vi "Fit N Gaussians.vi"(10 "Initial Parameters":T1(array[cluster]), 11 "Image In":T2) -> (0 "number of function calls":i32, 1 "Best-Fit Parameters":T1(array[cluster]), 2 "Best-Fit Image":T2, 3 "Image Src (Original)":T2)   [LabVIEW 2011]
uses:
  <vilib>/vision/Image Controls.llb/IMAQ Image.ctl
  <vilib>/gmath/NumericalOptimization/Nonlinear Curve Fit LM bound.vi
  <vilib>/gmath/NI_Gmath.lvlib
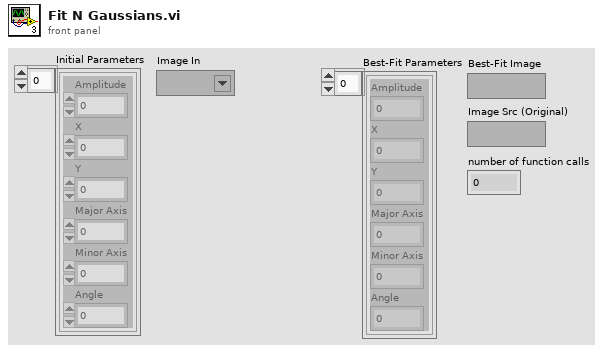
[diagram p1: front panel]
types:
  T1 = cluster{"Amplitude":dbl, "X":dbl, "Y":dbl, "Major Axis":dbl, "Minor Axis":dbl, "Angle":dbl}[]
  T2 = typedef "IMAQ Image.ctl" = refnum<image>
  T3 = typedef "Image Type" = u32
  T4 = cluster{"Width":i32, "Height":i32, "N Gaussians":i32}
  T5 = cluster{"Amplitude":dbl, "X":dbl, "Y":dbl, "Major Axis":dbl, "Minor Axis":dbl, "Angle":dbl}
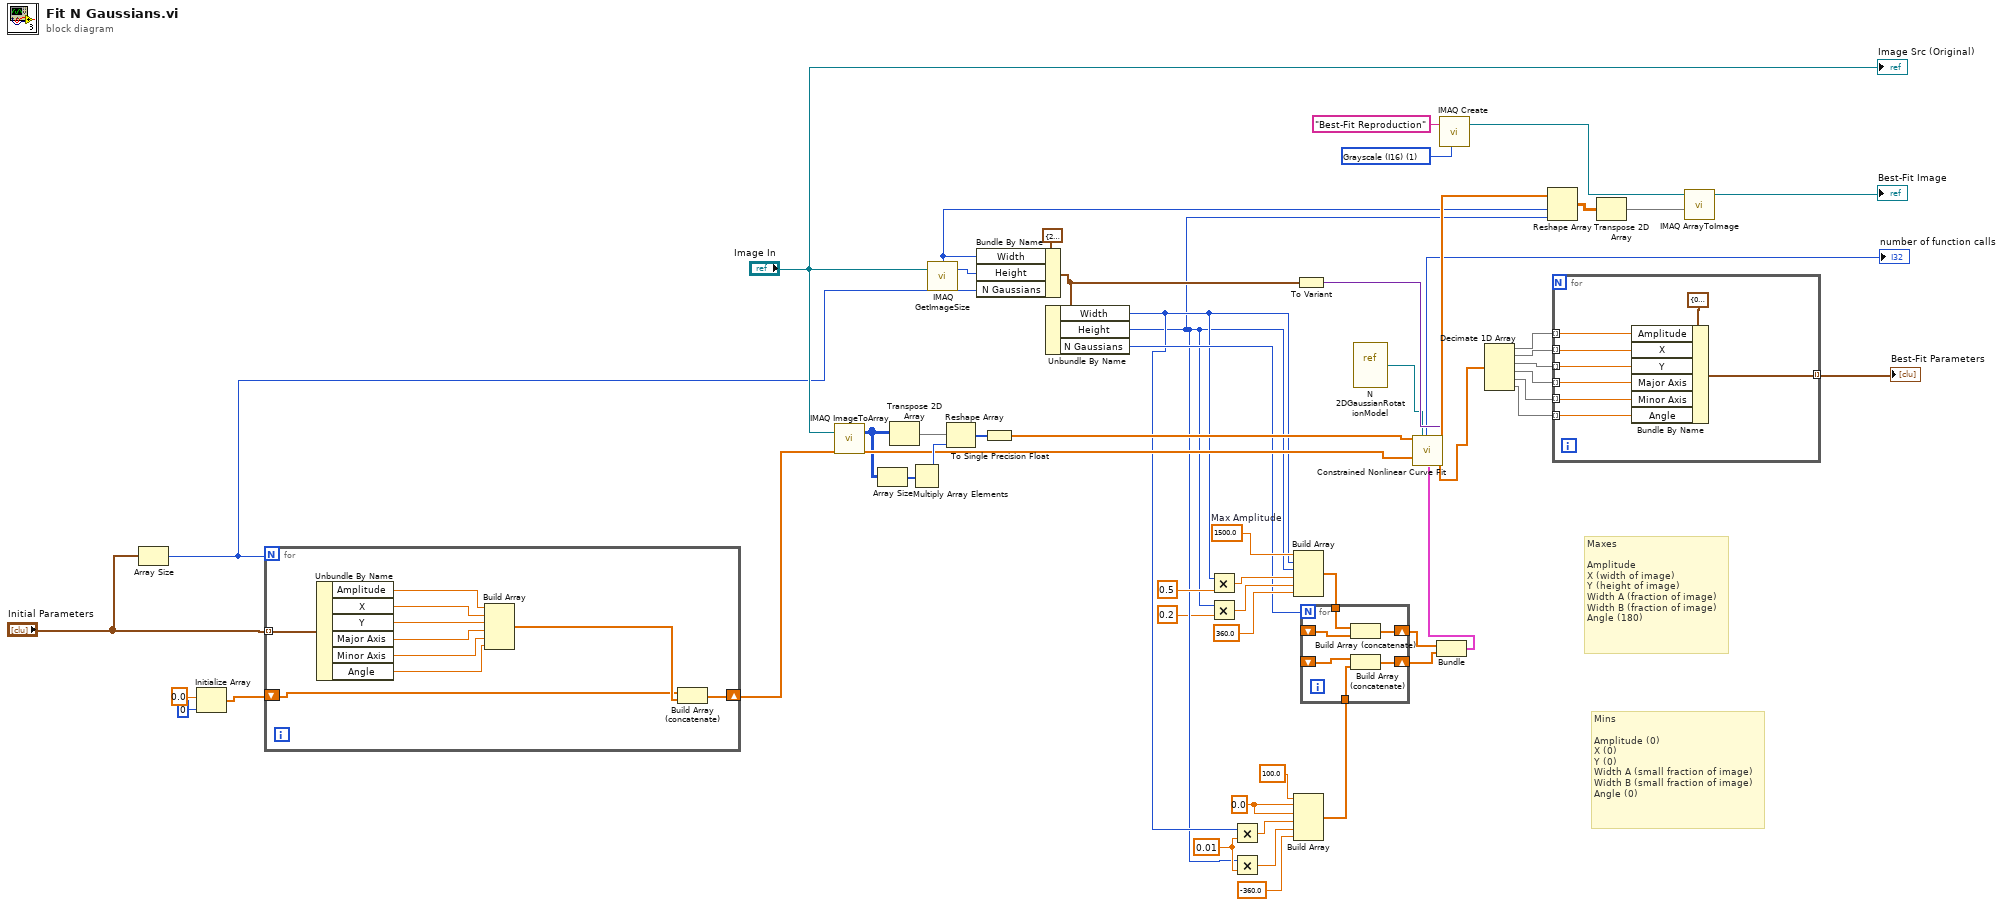
[diagram p0: block diagram]
diagram:
  w25 = 0.01
  w26 = 0.0 ("element")
  w32 = 1500.0  # Max Amplitude
  w43 = T3 1 items=["Grayscale (U8)", "Grayscale (I16)", "Grayscale (SGL)", "Complex (CSG)", "RGB (U32)", "HSL (U32)", "RGB (U64)", "Grayscale (U16)"] ("Image Type")
  # "Mins\n\nAmplitude (0)\nX (0)\nY (0)\nWidth A (small fraction of image)\nWidth B (small fraction of image)\nAngle (0)"
  # "Maxes\n\nAmplitude\nX (width of image)\nY (height of image)\nWidth A (fraction of image)\nWidth B (fraction of image)\nAngle (180)"
  n1 = Array Size(array="Initial Parameters") -> (size(s)=w15:i32)
  n2 = Initialize Array(0.0 ("element"), 0 ("dimension size")) -> (w4:dbl[])
  n3 = for {
    N: w15 -> [_]
    shift-right: [w64] -> w38
    shift-left: w4 -> [w63]
    tunnel: "Initial Parameters" -> [w62] mode=indexing
    n4 = Unbundle By Name(w62) -> ("Amplitude"=w61:dbl, "X"=w60:dbl, "Y"=w59:dbl, "Major Axis"=w58:dbl, "Minor Axis"=w57:dbl, "Angle"=w56:dbl)
    n5 = Build Array(w61, w60, w59, w58, w57, w56) -> (w65:dbl[])
    n6 = Build Array (concatenate)(w63, w65) -> (w64:dbl[])
  }
  n7 = call "IMAQ ImageToArray"("Image"="Image In") -> ("Image Pixels (I16)"=w9:i16[][])  [unwired: 3 in, 4 out]
  n8 = Array Size(array=w9) -> (size(s)=w53:i32[])
  n9 = Transpose 2D Array(2D array=w9) -> (transposed array=w8:i16[][])
  n10 = Multiply Array Elements(1:w53) -> (0:w54:i32)
  n11 = call "IMAQ GetImageSize"("Image"="Image In") -> ("Y Resolution"=w10:i32, "X Resolution"=w11:i32)  [unwired: 3 in, 1 out]
  n12 = Reshape Array(w8, w54) -> (w52:i16[])
  n13 = Bundle By Name(cluster=T4 {"Width"=25, "Height"=25, "N Gaussians"=2}, "Width"=w11, "Height"=w10, "N Gaussians"=w15) -> (w16:T4)
  n14 = To Single Precision Float(number=w52) -> (single precision float=w39:sgl[])
  n15 = Unbundle By Name(w16) -> ("Width"=w13:i32, "Height"=w12:i32, "N Gaussians"=w14:i32)
  n16 = Multiply(x=w13, y=0.5) -> (x*y=w30:dbl)
  n17 = Multiply(x=w12, y=0.2) -> (x*y=w29:dbl)
  n18 = Multiply(x=w13, y=w25) -> (x*y=w24:dbl)
  n19 = Multiply(x=w12, y=w25) -> (x*y=w23:dbl)
  n20 = Build Array(w32, w13, w12, w30, w29, 360.0 ("element")) -> (w21:dbl[])
  n21 = Build Array(100.0 ("element"), w26, w26, w24, w23, -360.0 ("element")) -> (w20:dbl[])
  n22 = To Variant(anything=w16) -> (Variant=w35:variant)
  n23 = for {
    N: w14 -> [_]
    shift-right: [w71] -> w19
    shift-left: _ -> [w66]
    tunnel: w21 -> [w70]
    tunnel: w20 -> [w68]
    shift-right: [w69] -> w18
    shift-left: _ -> [w67]
    n24 = Build Array (concatenate)(w70, w66) -> (w71:dbl[])
    n25 = Build Array (concatenate)(w67, w68) -> (w69:dbl[])
  }
  n26 = vi-ref "N 2DGaussianRotationModel.vi"() -> (w33:refnum<vi>)
  n27 = Bundle(w19, w18) -> (w17:cluster{dbl[], dbl[]})  [unwired: 1 in]
  n28 = call-poly <vilib>:"Constrained Nonlinear Curve Fit.vi"("Y"=w39, "f(x,a)"=w33, "data"=w35, "initial parameters"=w38, "parameter bounds"=w17) -> ("number of function calls"=→"number of function calls":i32, "best nonlinear fit"=w36:dbl[], "best fit parameters"=w37:dbl[])  [unwired: 5 in, 3 out]
  n29 = call "IMAQ Create"("Image Name"="Best-Fit Reproduction", "Image Type"=w43) -> ("New Image"=w42:T2)  [unwired: 3 in, 1 out]
  n30 = Decimate 1D Array(w37) -> (w51:dbl[], w50:dbl[], w49:dbl[], w48:dbl[], w47:dbl[], w46:dbl[])
  n31 = Reshape Array(w36, w11, w12) -> (w7:dbl[][])
  n32 = for {
    tunnel: w51 -> [w78] mode=indexing
    tunnel: w50 -> [w77] mode=indexing
    tunnel: w49 -> [w76] mode=indexing
    tunnel: w48 -> [w75] mode=indexing
    tunnel: w47 -> [w74] mode=indexing
    tunnel: w46 -> [w73] mode=indexing
    tunnel: [w72] -> w45 mode=indexing
    n33 = Bundle By Name(cluster=T5 {"Amplitude"=0.0, "X"=0.0, "Y"=0.0, "Major Axis"=0.0, "Minor Axis"=0.0, "Angle"=0.0}, "Amplitude"=w78, "X"=w77, "Y"=w76, "Major Axis"=w75, "Minor Axis"=w74, "Angle"=w73) -> (w72:T5)
  }
  "Best-Fit Parameters" <- w45
  n34 = Transpose 2D Array(2D array=w7) -> (transposed array=w6:dbl[][])
  n35 = call "IMAQ ArrayToImage"("Image Pixels (I16)"=w6, "Image"=w42) -> ("Image Out"=→"Best-Fit Image":T2)  [unwired: 8 in, 1 out]
  "Image Src (Original)" <- "Image In"
